vi "Set Pin Status.vi"(0 "NXP in":refnum<class "NXP.lvclass">, 5 "Port":dbl, 7 "Pin":dbl, 9 "Value":bool, 11 "error in (no error)":errorcluster) -> (4 "NXP out":refnum<class "NXP.lvclass">, 15 "error out":errorcluster)   [LabVIEW 2020, in "NXP.lvclass"]
uses:
  NXP.lvclass
  2aac738c-a9a9-47f1-a30e-954fde41d2a4.vi
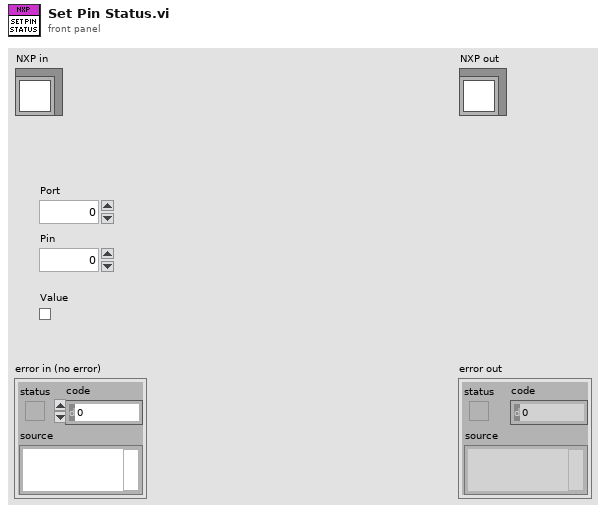
[diagram p1: front panel]
types:
  T1 = typedef "Serial device.lvclass/Brand combobox.ctl" = string
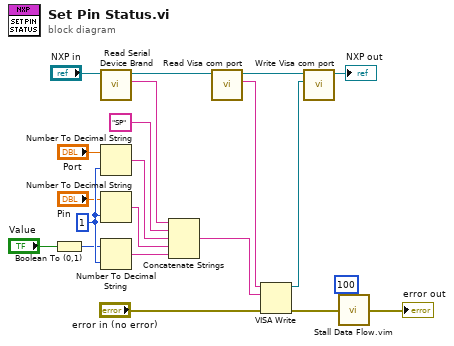
[diagram p0: block diagram]
diagram:
  w19 = i16 1 ("width (-)")
  n1 = Boolean To (0,1)(Boolean="Value") -> (0, 1=w18:i16)
  n2 = call-dynamic "Read Serial Device Brand.vi"("Serial device in"="NXP in") -> ("Serial Device Brand"=w14:T1, "Serial device out"=w20:refnum<class "NXP.lvclass">)  [unwired: 8 in, 1 out]
  n3 = Number To Decimal String(number="Port", width (-)=w19) -> (decimal integer string=w12:string)
  n4 = Number To Decimal String(number="Pin", width (-)=w19) -> (decimal integer string=w11:string)
  n5 = Number To Decimal String(number=w18, width (-)=w19) -> (decimal integer string=w10:string)
  n6 = Concatenate Strings(w14, "SP" ("string"), w12, w11, w10) -> (w9:string)
  n7 = call-dynamic "Read Visa com port.vi"("Serial device in"=w20) -> ("Visa com port"=w8:string, "Serial device out"=w5:refnum<class "NXP.lvclass">)  [unwired: 8 in, 1 out]
  n8 = VISA Write(VISA resource name=w8, write buffer=w9, error in (no error)="error in (no error)") -> (VISA resource name out=w3:refnum<visa-resource-name>, error out=w6:errorcluster)  [unwired: 1 out]
  n9 = call-dynamic "Write Visa com port.vi"("Visa com port"=w3, "Serial device in"=w5) -> ("Serial device out"=→"NXP out":refnum<class "NXP.lvclass">)  [unwired: 8 in, 1 out]
  n10 = call "Stall Data Flow.vim"("value in"=w6, "milliseconds to wait"=u32 100) -> ("value out"=→"error out":errorcluster)  [unwired: 1 out]
